vi "MU generate Biss Profile Id.vi"(8 "Error In":errorcluster, 10 "profile":u32, 11 "handle":u64) -> (0 "Error Out":errorcluster, 2 "bissProfileId":u16 format="%.0x", 3 "function return":u32)   [LabVIEW 2017, in "MU_3SL_interface.lvlib"]
uses:
  MU_3SL_interface.lvlib
  lib/MU_3SL_interface.dll
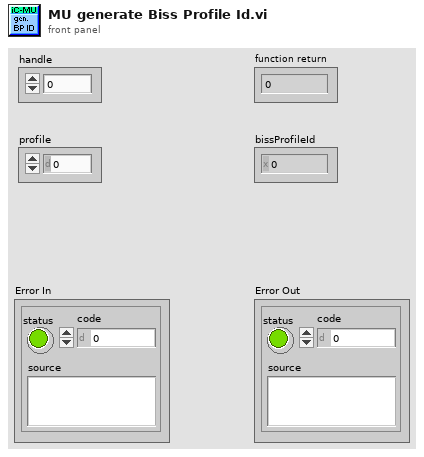
[diagram p1: front panel]
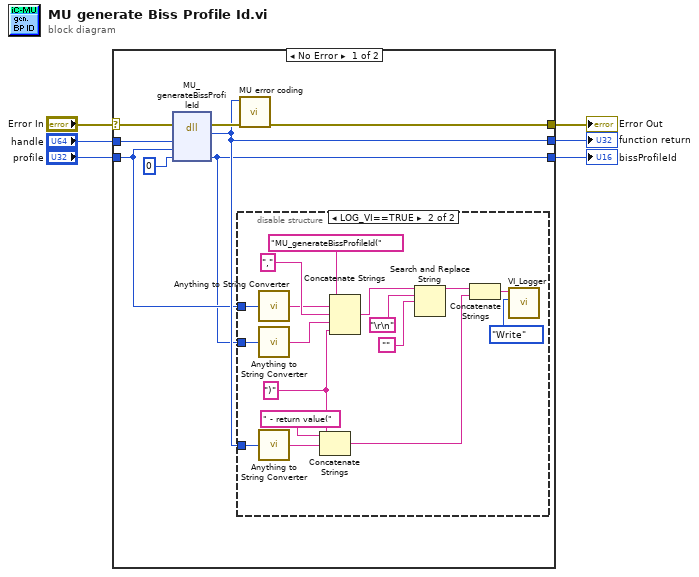
[diagram p0: block diagram]
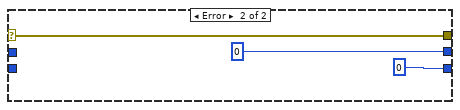
[diagram p3: hidden frame]
diagram:
  n1 = case shown="No Error" "Error In" {
    selector: "Error In" -> [w11 w34]
    tunnel: [w10 u32 0 ("return type")] -> w6
    tunnel: "handle" -> [w14 _]
    tunnel: [w12 w34] -> w4
    tunnel: [w7 u16 0 ("deviceID")] -> w2
    tunnel: "profile" -> [w8 _]
    frame No Error {
      n2 = dll-call lib="C:/Users/bes/AppData/Roaming/work/mu_9so/icsubmodules/soft_mu_3sl_master/lv_interface/lib/MU_3SL_interface**.*" fn="MU_generateBissProfileId"(error in=w11, "handle"=w14, "profile"=w8, "bissProfileId"=u16 0 ("mfgID")) -> (error out=w13:errorcluster, "return type"=w10:u32, "bissProfileId"=w7:u16)  [unwired: 4 in, 1 out]
      n3 = disable-structure shown="LOG_VI==TRUE" {
        disable-tunnel: w10 -> [_ w16]
        disable-tunnel: w8 -> [_ w18]
        disable-tunnel: w7 -> [_ w20]
        frame condition #0 {
        }
        frame condition #1 (active) {
          w26 = ")" ("string")
          n4 = call "Anything to String Converter.vi"("anything"=w18) -> ("String"=w17:string)
          n5 = call "Anything to String Converter.vi"("anything"=w20) -> ("String"=w19:string)
          n6 = call "Anything to String Converter.vi"("anything"=w16) -> ("String"=w15:string)
          n7 = Concatenate Strings(" - return value(" ("string"), w15, w26) -> (w29:string)
          n8 = Concatenate Strings("MU_generateBissProfileId(" ("Info in"), w17, "," ("string"), w19, w26) -> (w23:string)
          n9 = Search and Replace String(input string=w23, search string="\r\n", replace string="") -> (result string=w22:string)  [unwired: 5 in, 3 out]
          n10 = Concatenate Strings(w22, w29) -> (w28:string)
          n11 = call "VI_Logger.vi"("Action (Read)"=enum16{"Write", "Read"}."Write", "Info in"=w28) -> ()  [unwired: 8 in, 2 out]
        }
      }
      n12 = call "MU error coding.vi"("error in (no error)"=w13, "function return in"=w10) -> ("error out"=w12:errorcluster)  [unwired: 9 in]
    }
    frame Error {
    }
  }
  "function return" <- w6
  "Error Out" <- w4
  "bissProfileId" <- w2
